vi "VI Tree.vi"   [LabVIEW 2019, in "Minicircuit RF Switch Box.lvlib"]
doc: "This is the instrument driver for the <INSTRUMENT NAME>. The VI Tree displays all the user-callable VIs of the instrument driver in an organized table."
uses:
  <instrlib>/Minicircuit RF Switch Box/Minicircuit RF Switch Box.lvlib
panel:
  # "SEE DIAGRAM\nFOR VI TREE."
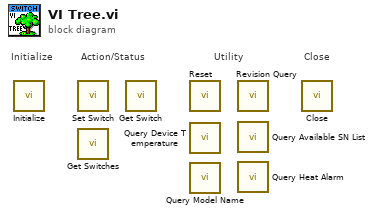
[diagram p0: block diagram]
diagram:
  # "Utility"
  # "Action/Status"
  # "Close"
  # "Initialize"
  n1 = call <instrlib>:"Initialize.vi"() -> ()  [unwired: 10 in, 2 out]
  n2 = call <instrlib>:"Set Switch.vi"() -> ()  [unwired: 10 in, 2 out]
  n3 = call <instrlib>:"Get Switches.vi"() -> ()  [unwired: 9 in, 3 out]
  n4 = call <instrlib>:"Get Switch.vi"() -> ()  [unwired: 9 in, 3 out]
  n5 = call <instrlib>:"Reset.vi"() -> ()  [unwired: 10 in, 2 out]
  n6 = call <instrlib>:"Query Device T emperature.vi"() -> ()  [unwired: 9 in, 3 out]
  n7 = call <instrlib>:"Query Model Name.vi"() -> ()  [unwired: 9 in, 3 out]
  n8 = call <instrlib>:"Revision Query.vi"() -> ()  [unwired: 8 in, 4 out]
  n9 = call <instrlib>:"Query Available SN List.vi"() -> ()  [unwired: 9 in, 3 out]
  n10 = call <instrlib>:"Query Heat Alarm.vi"() -> ()  [unwired: 9 in, 3 out]
  n11 = call <instrlib>:"Close.vi"() -> ()  [unwired: 11 in, 1 out]
